vi "test vi.vi"   [LabVIEW 2015]
uses:
  <vilib>/Utility/config.llb/NI_LVConfig.lvlib
types:
  T1 = typedef "NI_LVConfig.lvlib/Config Data RefNum.ctl" = refnum<k1>
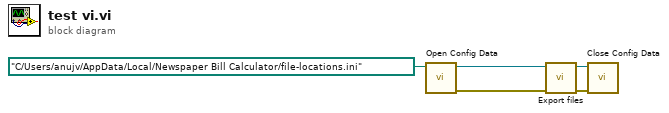
[diagram p0: block diagram]
diagram:
  n1 = call <vilib>:"Open Config Data.vi"("configuration file path"=path "C:/Users/anujv/AppData/Local/Newspaper Bill Calculator/file-locations.ini") -> ("error out"=w3:errorcluster, "refnum"=w4:T1)  [unwired: 8 in, 1 out]
  n2 = call "Export files.vi"("Error In"=w3, "INI ref in"=w4) -> ("Error Out"=w1:errorcluster, "INI ref out"=w2:T1)  [unwired: 8 in]
  n3 = call <vilib>:"Close Config Data.vi"("error in (no error)"=w1, "refnum"=w2) -> ()  [unwired: 8 in, 2 out]
